vi "Query ID.vi"(8 "error in (no error)":errorcluster, 10 "Query String(*IDN?)":string="*IDN?", 11 "DMM in":refnum<class "CS Emulation.lvclass">) -> (0 "error out":errorcluster, 2 "ID  string":string, 3 "DMM out":refnum<class "CS Emulation.lvclass">)   [LabVIEW 2016, in "CS Emulation.lvclass"]
uses:
  Lib.llb/CS Emulation.lvclass
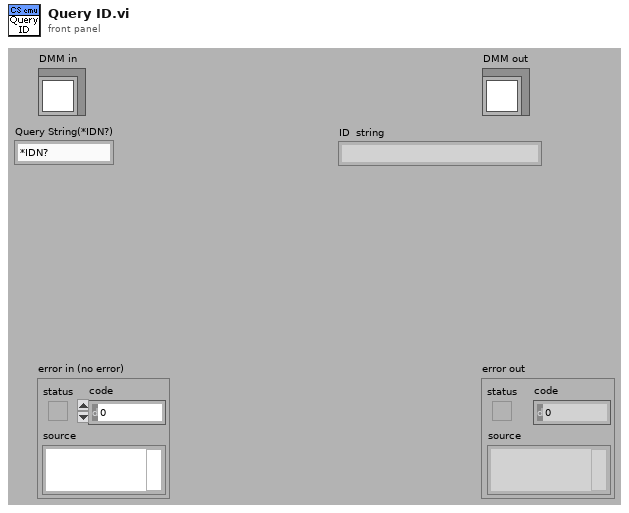
[diagram p1: front panel]
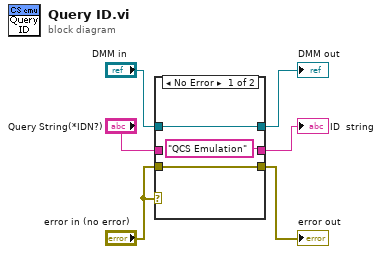
[diagram p0: block diagram]
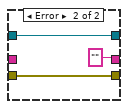
[diagram p2: hidden frame]
diagram:
  n1 = case shown="No Error" "error in (no error)" {
    tunnel: [w8 w12] -> w6
    tunnel: ["QCS Emulation" ("ID  string") "" ("ID  string")] -> w5
    tunnel: [w9 w11] -> w4
    tunnel: "error in (no error)" -> [w8 w12]
    tunnel: "Query String(*IDN?)" -> [_ _]
    tunnel: "DMM in" -> [w9 w11]
    frame No Error {
    }
    frame Error {
    }
  }
  "error out" <- w6
  "DMM out" <- w4
  "ID  string" <- w5
